vi "Calculate Normal Array.vi"(8 "error in (no error)":errorcluster, 9 "Coordinates System":enum16{"Cartesian", "Cylindrical", "Spherical"}(ring), 10 "3D Pie Datatype.lvclass in":refnum<class "3D Pie Datatype.lvclass">, 11 "Plot Representation In":T1) -> (0 "error out":errorcluster, 1 "Dup Coordinates System":enum16{"Cartesian", "Cylindrical", "Spherical"}(ring), 2 "3D Pie Datatype.lvclass out":refnum<class "3D Pie Datatype.lvclass">, 3 "Plot Representation Out":T1)   [LabVIEW 2020, in "3D Pie Datatype.lvclass"]
uses:
  <vilib>/Math Plots/3D Math Plots/3D Pie/3D Pie Datatype/3D Pie Datatype.lvclass
  <vilib>/Math Plots/3D Math Plots/3D Plot/3D Plot/Typedef/Plot Representation.ctl
  <vilib>/Math Plots/3D Math Plots/3D Plot/3D Plot/Typedef/Range Clusters.ctl
  <vilib>/Math Plots/3D Math Plots/3D Plot/3D Plot/Typedef/Mesh Data.ctl
  <vilib>/Math Plots/3D Math Plots/3D Pie/3D Pie Datatype/3D Pie Datatype.lvclass/3D Pie Datatype.ctl
  <vilib>/Math Plots/3D Math Plots/3D Plot/3D Plot/3D Plot.lvclass
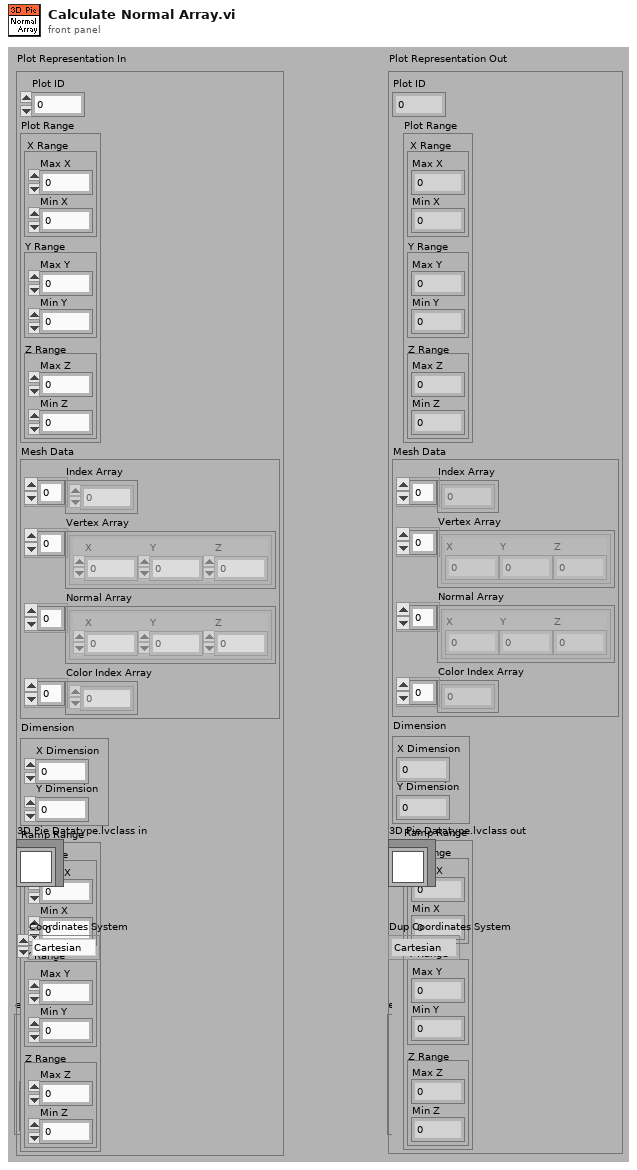
[diagram p1: front panel]
types:
  T1 = typedef "3D Plot.lvclass/Plot Representation.ctl" = cluster{"Plot ID":i32, "Plot Range":T2, "Mesh Data":T3, "Dimension":cluster{"X Dimension":i32, "Y Dimension":i32}, "Ramp Range":T2}
  T2 = typedef "3D Plot.lvclass/Range Clusters.ctl" = cluster{"X Range":cluster{"Max X":sgl, "Min X":sgl}, "Y Range":cluster{"Max Y":sgl, "Min Y":sgl}, "Z Range":cluster{"Max Z":sgl, "Min Z":sgl}}
  T3 = typedef "3D Plot.lvclass/Mesh Data.ctl" = cluster{"Index Array":u32[], "Vertex Array":cluster{"X":sgl, "Y":sgl, "Z":sgl}[], "Normal Array":cluster{"X":sgl, "Y":sgl, "Z":sgl}[], "Color Index Array":i32[]}
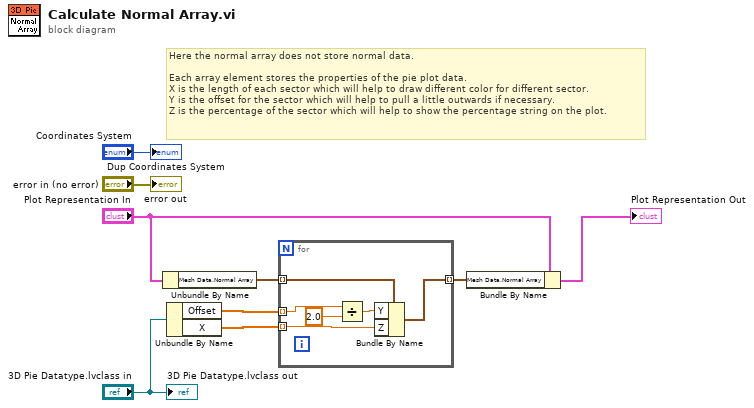
[diagram p0: block diagram]
diagram:
  # "Here the normal array does not store normal data.\n\nEach array element stores the properties of the pie plot data.\nX is the length of each sector which will help to draw different color for different sector.\nY is the offset for the sector which will help to pull a little outwards if necessary.\nZ is the percentage of the sector which will help to show the percentage string on the plot."
  n1 = Unbundle By Name("Plot Representation In") -> ("Mesh Data.Normal Array"=w2:cluster{"X":sgl, "Y":sgl, "Z":sgl}[])
  n2 = Unbundle By Name("3D Pie Datatype.lvclass in") -> ("Offset"=w3:sgl[], "X"=w1:sgl[])
  n3 = for {
    tunnel: w3 -> [w11] mode=indexing
    tunnel: [w14] -> w4 mode=indexing
    tunnel: w1 -> [w10] mode=indexing
    tunnel: w2 -> [w15] mode=indexing
    n4 = Divide(x=w11, y=sgl 2.0) -> (x/y=w12:sgl)
    n5 = Bundle By Name(cluster=w15, "Y"=w12, "Z"=w10) -> (w14:cluster{"X":sgl, "Y":sgl, "Z":sgl})
  }
  n6 = Bundle By Name(cluster="Plot Representation In", "Mesh Data.Normal Array"=w4) -> (→"Plot Representation Out":T1)
  "error out" <- "error in (no error)"
  "3D Pie Datatype.lvclass out" <- "3D Pie Datatype.lvclass in"
  "Dup Coordinates System" <- "Coordinates System"
